vi "Create 2 In 2 Out DRAM Resources.vi"(0 "common resources":T11={"sync pulse resources"={"sync pulse destination terminal"="", "sync100"="", "sync pulse source terminal"="", "imported sync pulse register"="", "generate sync pulse handshake"="", "enable sync pulse register"="", "sync pulse clock"=""}, "serial channel resources"={"sc 0"={"completed frames register"=""}, "sc 1"={"completed frames register"=""}, "sc 2"={"completed frames register"=""}, "sc 3"={"completed frames register"=""}, "sc 4"={"completed frames register"=""}, "sc 5"={"completed frames register"=""}, "sc 6"={"completed frames register"=""}, "sc 7"={"completed frames register"=""}}, "dram manager 0"={"DRAM class"=refnum, "process clock"="", "registers"={"configuration"={"write time slice"="", "request time slice"="", "DRAM arbiter config"="", "partition config"=""}, "reset"={"handshake"={"start.go"="", "start.go rcvd"="", "done.go"="", "done.go rcvd"=""}, "process"={"in"="", "out"=""}, "write"={"in"="", "out 0"="", "out 1"="", "out 2"="", "out 3"=""}, "read"={"in"="", "out 0"="", "out 1"="", "out 2"="", "out 3"=""}}, "status"={"partition full"=""}}, "FIFOs"={"write data"={"FIFO 0"="", "FIFO 1"="", "FIFO 2"="", "FIFO 3"=""}, "request metadata"={"FIFO"=""}, "read data VOQ"={"FIFO 0"="", "FIFO 1"="", "FIFO 2"="", "FIFO 3"=""}, "read data"={"FIFO 0"="", "FIFO 1"="", "FIFO 2"="", "FIFO 3"=""}}, "num active streams"=0.0, "max open read requests"=256}, "dram manager 1"={"DRAM class"=refnum, "process clock"="", "registers"={"configuration"={"write time slice"="", "request time slice"="", "DRAM arbiter config"="", "partition config"=""}, "reset"={"handshake"={"start.go"="", "start.go rcvd"="", "done.go"="", "done.go rcvd"=""}, "process"={"in"="", "out"=""}, "write"={"in"="", "out 0"="", "out 1"="", "out 2"="", "out 3"=""}, "read"={"in"="", "out 0"="", "out 1"="", "out 2"="", "out 3"=""}}, "status"={"partition full"=""}}, "FIFOs"={"write data"={"FIFO 0"="", "FIFO 1"="", "FIFO 2"="", "FIFO 3"=""}, "request metadata"={"FIFO"=""}, "read data VOQ"={"FIFO 0"="", "FIFO 1"="", "FIFO 2"="", "FIFO 3"=""}, "read data"={"FIFO 0"="", "FIFO 1"="", "FIFO 2"="", "FIFO 3"=""}}, "num active streams"=0.0, "max open read requests"=256}}, 5 "dram partition configs":T10[](array[typedef])=[{"first address"=0, "last address"=0}, {"first address"=0, "last address"=0}, {"first address"=0, "last address"=0}, {"first address"=0, "last address"=0}, {"first address"=0, "last address"=0}, {"first address"=0, "last address"=0}, {"first address"=0, "last address"=0}, {"first address"=0, "last address"=0}]) -> (4 "channel dram resources":T1)   [LabVIEW 2020, in "GettingStarted_Gen_148X_FPGA.lvlib"]
uses:
  GettingStarted_Gen_148X_FPGA.lvlib
  Common/Types/Common Resources.ctl
  <instrlib>/_niInstr/Memory/v1/FPGA/DRAM/niInstr Memory DRAM v1 FPGA.lvclass
  <instrlib>/FlexRIO/CSI-2/v2/FPGA/Types/Sync Pulse Resources.ctl
  Common/Types/Serial Channel Resources.ctl
  Common/Types/Single Serial Channel Resources.ctl
  <instrlib>/FlexRIO/CSI-2/v2/FPGA/DRAM Manager/Private/DRAM Manager.ctl
  <instrlib>/FlexRIO/CSI-2/v2/FPGA/DRAM Manager/Private/Common/DRAM Manager Registers.ctl
  <instrlib>/FlexRIO/CSI-2/v2/FPGA/DRAM Manager/Private/Common/Handshake Registers.ctl
  <instrlib>/FlexRIO/CSI-2/v2/FPGA/DRAM Manager/Private/Common/DRAM Manager FIFOs.ctl
  <instrlib>/FlexRIO/CSI-2/v2/FPGA/DRAM Manager/Private/Common/Write Data FIFO Ref.ctl
  <instrlib>/FlexRIO/CSI-2/v2/FPGA/DRAM Manager/Private/Common/Read Request Metadata FIFO Ref.ctl
  <instrlib>/FlexRIO/CSI-2/v2/FPGA/DRAM Manager/Private/Common/Read Data FIFO Ref.ctl
  <instrlib>/FlexRIO/CSI-2/v2/FPGA/DRAM Manager/Public/Partition Range.ctl
  Types/2 In 2 Out DRAM Resources.ctl
  Types/Serial Output DRAM Resources.ctl
  <instrlib>/FlexRIO/CSI-2/v2/FPGA/DRAM Manager/DRAM Manager v2.lvlib
  <instrlib>/FlexRIO/CSI-2/v2/FPGA/NI CSI-2 API FPGA v2.lvlib
  Common/GettingStarted_Common_148X_FPGA.lvlib
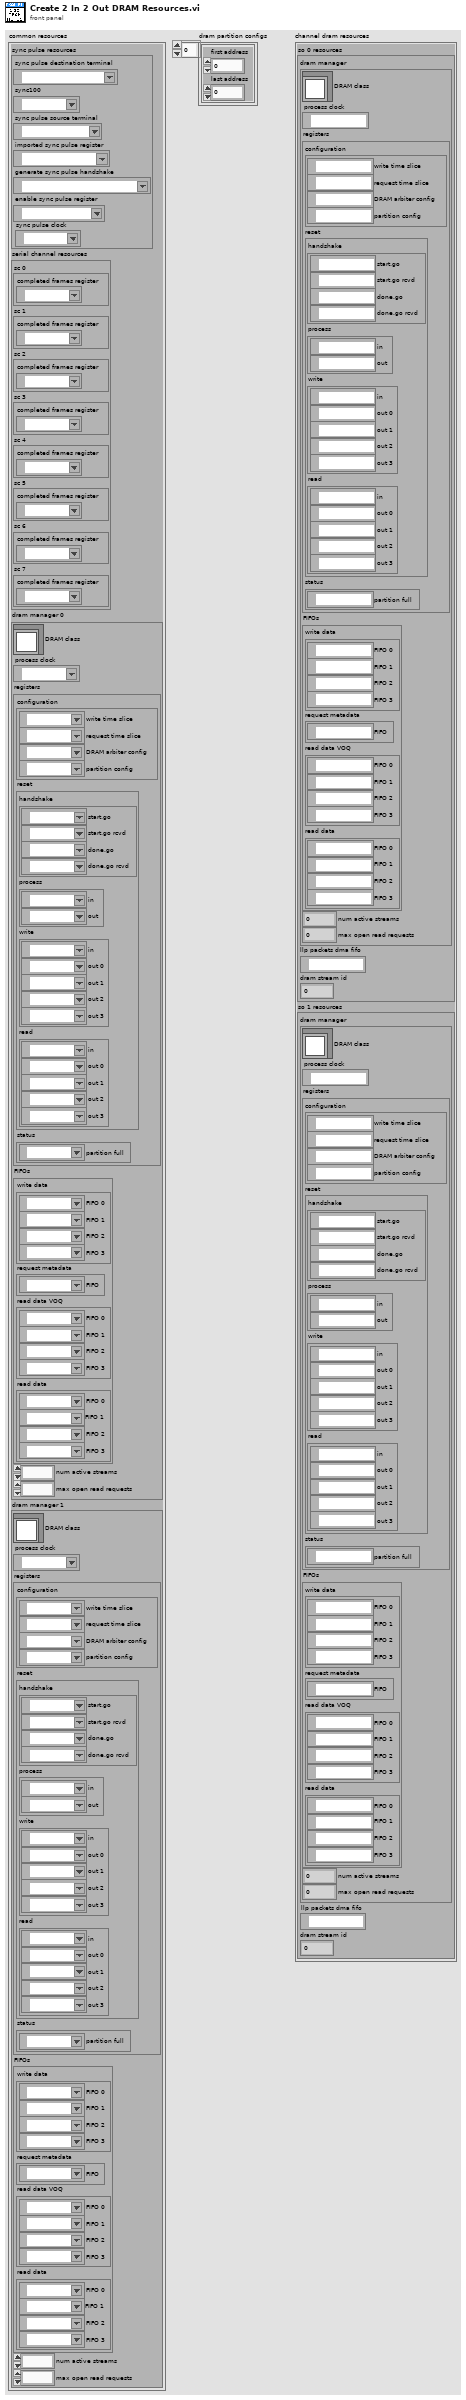
[diagram p1: front panel]
types:
  T1 = typedef "GettingStarted_Gen_148X_FPGA.lvlib/2 In 2 Out DRAM Resources.ctl" = cluster{"so 0 resources":T2, "so 1 resources":T2}
  T2 = typedef "GettingStarted_Gen_148X_FPGA.lvlib/Serial Output DRAM Resources.ctl" = cluster{"dram manager":T3, "llp packets dma fifo":refnum<k21>, "dram stream id":fxp<+,2,2>}
  T3 = typedef "DRAM Manager v2.lvlib/DRAM Manager.ctl" = cluster{"DRAM class":refnum<class "niInstr Memory DRAM v1 FPGA.lvclass">, "process clock":refnum<k21>, "registers":T4, "FIFOs":T6, "num active streams":fxp<+,3,3>, "max open read requests":u16}
  T4 = typedef "DRAM Manager v2.lvlib/DRAM Manager Registers.ctl" = cluster{"configuration":cluster{"write time slice":refnum<k21>, "request time slice":refnum<k21>, "DRAM arbiter config":refnum<k21>, "partition config":refnum<k21>}, "reset":cluster{"handshake":T5, "process":cluster{"in":refnum<k21>, "out":refnum<k21>}, "write":cluster{"in":refnum<k21>, "out 0":refnum<k21>, "out 1":refnum<k21>, "out 2":refnum<k21>, "out 3":refnum<k21>}, "read":cluster{"in":refnum<k21>, "out 0":refnum<k21>, "out 1":refnum<k21>, "out 2":refnum<k21>, "out 3":refnum<k21>}}, "status":cluster{"partition full":refnum<k21>}}
  T5 = typedef "DRAM Manager v2.lvlib/Handshake Registers.ctl" = cluster{"start.go":refnum<k21>, "start.go rcvd":refnum<k21>, "done.go":refnum<k21>, "done.go rcvd":refnum<k21>}
  T6 = typedef "DRAM Manager v2.lvlib/DRAM Manager FIFOs.ctl" = cluster{"write data":cluster{"FIFO 0":T7, "FIFO 1":T7, "FIFO 2":T7, "FIFO 3":T7}, "request metadata":cluster{"FIFO":T8}, "read data VOQ":cluster{"FIFO 0":T9, "FIFO 1":T9, "FIFO 2":T9, "FIFO 3":T9}, "read data":cluster{"FIFO 0":T9, "FIFO 1":T9, "FIFO 2":T9, "FIFO 3":T9}}
  T7 = typedef "DRAM Manager v2.lvlib/Write Data FIFO Ref.ctl" = refnum<k21>
  T8 = typedef "DRAM Manager v2.lvlib/Read Request Metadata FIFO Ref.ctl" = refnum<k21>
  T9 = typedef "DRAM Manager v2.lvlib/Read Data FIFO Ref.ctl" = refnum<k21>
  T10 = typedef "DRAM Manager v2.lvlib/Partition Range.ctl" = cluster{"first address":u32, "last address":u32}
  T11 = typedef "GettingStarted_Common_148X_FPGA.lvlib/Common Resources.ctl" = cluster{"sync pulse resources":T12, "serial channel resources":T13, "dram manager 0":T3, "dram manager 1":T3}
  T12 = typedef "NI CSI-2 API FPGA v2.lvlib/Sync Pulse Resources.ctl" = cluster{"sync pulse destination terminal":refnum<k21>, "sync100":refnum<k21>, "sync pulse source terminal":refnum<k21>, "imported sync pulse register":refnum<k21>, "generate sync pulse handshake":refnum<k21>, "enable sync pulse register":refnum<k21>, "sync pulse clock":refnum<k21>}
  T13 = typedef "GettingStarted_Common_148X_FPGA.lvlib/Serial Channel Resources.ctl" = cluster{"sc 0":T14, "sc 1":T14, "sc 2":T14, "sc 3":T14, "sc 4":T14, "sc 5":T14, "sc 6":T14, "sc 7":T14}
  T14 = typedef "GettingStarted_Common_148X_FPGA.lvlib/Single Serial Channel Resources.ctl" = cluster{"completed frames register":refnum<k21>}
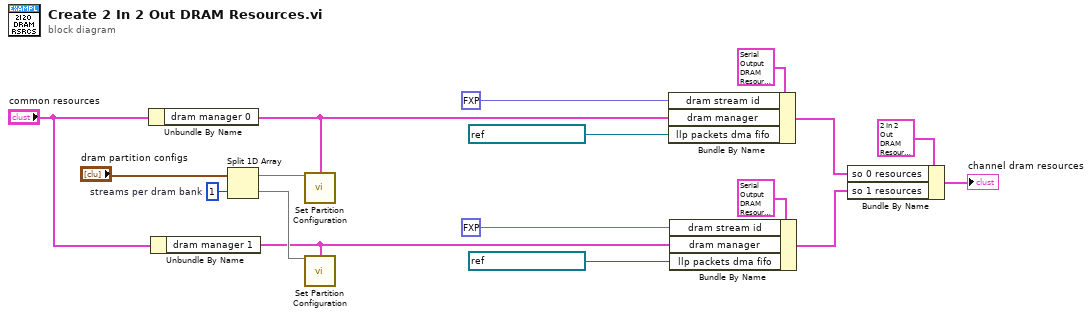
[diagram p0: block diagram]
diagram:
  w12 = 1  # streams per dram bank
  n1 = Unbundle By Name("common resources") -> ("dram manager 0"=w5:T3)
  n2 = Unbundle By Name("common resources") -> ("dram manager 1"=w4:T3)
  n3 = Split 1D Array(array="dram partition configs", index=w12) -> (first subarray=w13:T10[], second subarray=w11:T10[])
  n4 = call <instrlib>:"Set Partition Configuration.vi"("partition config"=w13, "DRAM manager"=w5) -> ()  [unwired: 14 in]
  n5 = call <instrlib>:"Set Partition Configuration.vi"("partition config"=w11, "DRAM manager"=w4) -> ()  [unwired: 14 in]
  n6 = Bundle By Name(cluster=T2 {"dram manager"={"DRAM class"=refnum, "process clock"="", "registers"={"configuration"={"write time slice"="", "request time slice"="", "DRAM arbiter config"="", "partition config"=""}, "reset"={"handshake"={"start.go"="", "start.go rcvd"="", "done.go"="", "done.go rcvd"=""}, "process"={"in"="", "out"=""}, "write"={"in"="", "out 0"="", "out 1"="", "out 2"="", "out 3"=""}, "read"={"in"="", "out 0"="", "out 1"="", "out 2"="", "out 3"=""}}, "status"={"partition full"=""}}, "FIFOs"={"write data"={"FIFO 0"="", "FIFO 1"="", "FIFO 2"="", "FIFO 3"=""}, "request metadata"={"FIFO"=""}, "read data VOQ"={"FIFO 0"="", "FIFO 1"="", "FIFO 2"="", "FIFO 3"=""}, "read data"={"FIFO 0"="", "FIFO 1"="", "FIFO 2"="", "FIFO 3"=""}}, "num active streams"=0.0, "max open read requests"=0}, "llp packets dma fifo"="", "dram stream id"=0.0} ("resources"), "dram stream id"=fxp<+,2,2> 0.0, "dram manager"=w5, "llp packets dma fifo"=refnum<k21> "SO 0 LLP Packets" ("llp data dma fifo")) -> (w16:T2)
  n7 = Bundle By Name(cluster=T2 {"dram manager"={"DRAM class"=refnum, "process clock"="", "registers"={"configuration"={"write time slice"="", "request time slice"="", "DRAM arbiter config"="", "partition config"=""}, "reset"={"handshake"={"start.go"="", "start.go rcvd"="", "done.go"="", "done.go rcvd"=""}, "process"={"in"="", "out"=""}, "write"={"in"="", "out 0"="", "out 1"="", "out 2"="", "out 3"=""}, "read"={"in"="", "out 0"="", "out 1"="", "out 2"="", "out 3"=""}}, "status"={"partition full"=""}}, "FIFOs"={"write data"={"FIFO 0"="", "FIFO 1"="", "FIFO 2"="", "FIFO 3"=""}, "request metadata"={"FIFO"=""}, "read data VOQ"={"FIFO 0"="", "FIFO 1"="", "FIFO 2"="", "FIFO 3"=""}, "read data"={"FIFO 0"="", "FIFO 1"="", "FIFO 2"="", "FIFO 3"=""}}, "num active streams"=0.0, "max open read requests"=0}, "llp packets dma fifo"="", "dram stream id"=0.0} ("resources"), "dram stream id"=fxp<+,2,2> 0.0, "dram manager"=w4, "llp packets dma fifo"=refnum<k21> "SO 1 LLP Packets" ("llp data dma fifo")) -> (w1:T2)
  n8 = Bundle By Name(cluster=T1 {"so 0 resources"={"dram manager"={"DRAM class"=refnum, "process clock"="", "registers"={"configuration"={"write time slice"="", "request time slice"="", "DRAM arbiter config"="", "partition config"=""}, "reset"={"handshake"={"start.go"="", "start.go rcvd"="", "done.go"="", "done.go rcvd"=""}, "process"={"in"="", "out"=""}, "write"={"in"="", "out 0"="", "out 1"="", "out 2"="", "out 3"=""}, "read"={"in"="", "out 0"="", "out 1"="", "out 2"="", "out 3"=""}}, "status"={"partition full"=""}}, "FIFOs"={"write data"={"FIFO 0"="", "FIFO 1"="", "FIFO 2"="", "FIFO 3"=""}, "request metadata"={"FIFO"=""}, "read data VOQ"={"FIFO 0"="", "FIFO 1"="", "FIFO 2"="", "FIFO 3"=""}, "read data"={"FIFO 0"="", "FIFO 1"="", "FIFO 2"="", "FIFO 3"=""}}, "num active streams"=0.0, "max open read requests"=0}, "llp packets dma fifo"="", "dram stream id"=0.0}, "so 1 resources"={"dram manager"={"DRAM class"=refnum, "process clock"="", "registers"={"configuration"={"write time slice"="", "request time slice"="", "DRAM arbiter config"="", "partition config"=""}, "reset"={"handshake"={"start.go"="", "start.go rcvd"="", "done.go"="", "done.go rcvd"=""}, "process"={"in"="", "out"=""}, "write"={"in"="", "out 0"="", "out 1"="", "out 2"="", "out 3"=""}, "read"={"in"="", "out 0"="", "out 1"="", "out 2"="", "out 3"=""}}, "status"={"partition full"=""}}, "FIFOs"={"write data"={"FIFO 0"="", "FIFO 1"="", "FIFO 2"="", "FIFO 3"=""}, "request metadata"={"FIFO"=""}, "read data VOQ"={"FIFO 0"="", "FIFO 1"="", "FIFO 2"="", "FIFO 3"=""}, "read data"={"FIFO 0"="", "FIFO 1"="", "FIFO 2"="", "FIFO 3"=""}}, "num active streams"=0.0, "max open read requests"=0}, "llp packets dma fifo"="", "dram stream id"=0.0}} ("2 in 2 out dram resources"), "so 0 resources"=w16, "so 1 resources"=w1) -> (→"channel dram resources":T1)
